vi "fgv_state-machine_config.vi"(7 "cmd":enum16{"write", "read"}(ring), 11 "Angle cfg":T1={" turn angular speed"=0.5, "move linear speed"=0.5, "decrease factor linear speed"=80.0, "adjust angle margin"=9.0} {"decrease factor linear speed" min=1.0}) -> (3 "Angle cfg out":T1={" turn angular speed"=0.5, "move linear speed"=0.5, "decrease factor linear speed"=80.0, "adjust angle margin"=9.0})   [LabVIEW 2019]
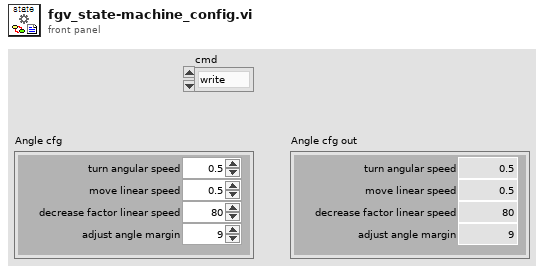
[diagram p1: front panel]
types:
  T1 = cluster{" turn angular speed":dbl, "move linear speed":dbl, "decrease factor linear speed":dbl, "adjust angle margin":dbl}
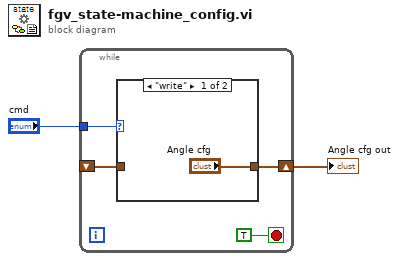
[diagram p0: block diagram]
diagram:
  n1 = while {
    tunnel: "cmd" -> [w5]
    shift-right: [w4] -> w1
    shift-left: _ -> [w3]
    stop <- TRUE stop-if-true
    n2 = case shown="\"write\"" w5 {
      tunnel: ["Angle cfg" w8] -> w4
      tunnel: w3 -> [_ w8]
      frame "write" {
      }
      frame "read", Default {
      }
    }
  }
  "Angle cfg out" <- w1
